vi "acender_boolean_push_button.vi"() -> ()   [LabVIEW 2018]
uses:
  <vilib>/Instr/_visa.llb/VISA Configure Serial Port (Instr).vi
panel:
  out "Boolean":bool
  in  "VISA resource name":refnum<visa-resource-name>
  in  "stop":bool
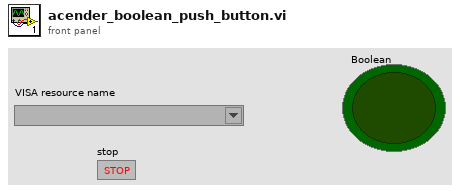
[diagram p1: front panel]
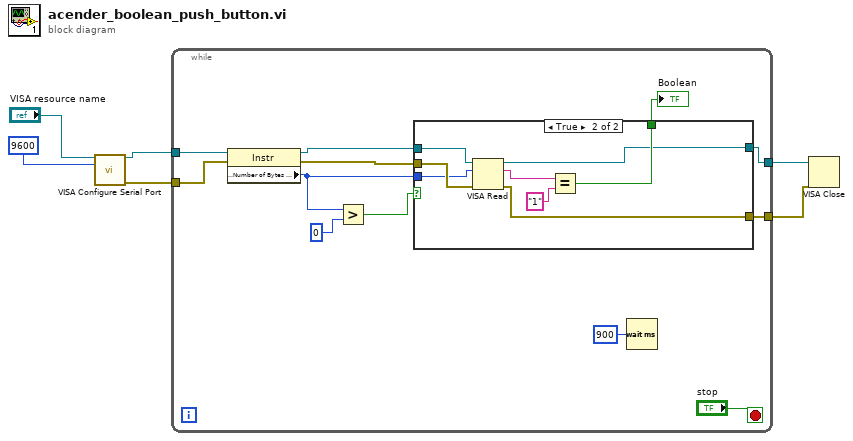
[diagram p0: block diagram]
diagram:
  n1 = call-poly "VISA Configure Serial Port"("VISA resource name"="VISA resource name", "baud rate (9600)"=u32 9600) -> ("VISA resource name out"=w6:refnum<visa-resource-name>, "error out"=w5:errorcluster)  [unwired: 12 in]
  n2 = while {
    tunnel: w6 -> [w15]
    tunnel: w5 -> [w14]
    tunnel: [w8] -> w2
    tunnel: [w7] -> w1
    stop <- "stop" stop-if-true
    n3 = property class="Instr"(reference=w15, error in=w14) -> (reference out=w13:refnum<visa-resource-name>, error out=w11:errorcluster, "Serial Settings:Number of Bytes at Serial Port"=w10:u32)
    n4 = Greater?(x=w10, y=u32 0) -> (0:w12:bool)
    n5 = case shown="True" w12 {
      tunnel: w13 -> [w20 w28]
      tunnel: w11 -> [w19 w27]
      tunnel: w10 -> [_ w26]
      tunnel: [_ w23] -> w9
      tunnel: [w20 w22] -> w8
      tunnel: [w19 w21] -> w7
      frame False {
      }
      frame True {
        n6 = VISA Read(VISA resource name=w28, byte count=w26, error in (no error)=w27) -> (VISA resource name out=w22:refnum<visa-resource-name>, read buffer=w25:string, error out=w21:errorcluster)  [unwired: 1 out]
        n7 = Equal?(x=w25, y="1") -> (x = y?=w23:bool)
      }
    }
    "Boolean" <- w9
    n8 = Wait (ms)(milliseconds to wait=u32 900) -> ()  [unwired: 1 out]
  }
  n9 = VISA Close(VISA resource name=w2, error in (no error)=w1) -> ()  [unwired: 1 out]
